vi "sv_STFT by Increment.vi"(0 "scaled signal [EU]":waveform(dbl), 1 "weighting filter":T5 items=["Linear", "A-weighting", "B-weighting", "C-weighting", "ITU-R 468-4", "Dolby", "CCITT", "C-message", "Wb", "Wc", "Wd", "We", "Wf", "Wh", "Wj", "Wk", "Wm", "AES17 20 kHz lowpass", "AES17 40 kHz lowpass", "AES17 20 kHz highpass", "AES17 40 kHz highpass"], 7 "FFT info":T7={"FFT block size"=1024, "number of FFT"=0, "start index"=0, "increment"=0.0} {"increment" format="%.2f"}, 11 "error in (no error)":errorcluster, 12 "window":T8(ring)=enum."Hanning", 13 "dB On (T)":bool=TRUE) -> (4 "power spectra [dB EU]":dbl[][](array[numeric]) format="%.2f", 6 "unit label":string, 8 "f0 and delta f [Hz]":cluster{"f0":dbl, "delta f":dbl} {"delta f" format="%.2f"; "f0" format="%.2f"}, 10 "spectrum info":T1={"channel name"="", "description"="", "x-axis units"=0, "spectral info"={"spectrum type"=enum."Power [Magnitude^2]", "linear/dB"=enum."linear", "window"=0, "window size"=0, "FFT size"=0}, "engineering units"=0, "custom label"="", "dB reference [EU]"=0.0, "peak units"=enum."rms", "weighting filter"=0, "spectral density?"=FALSE, "unit label"="", "spectrum skewed?"=FALSE, "complimentary spectrum units"=enum."none"} {"x-axis units" items=["Time (s)"=0, "Frequency-CB (Hz)"=1, "Frequency-CPB (Hz)"=1248, "Frequency-Arbitrary (Hz)"=2357, "Quefrency (s)"=2, "Revolutions (rev)"=3, "Order"=4, "Speed (RPM)"=11, "Speed (rad/s)"=21, "Index"=65535]; "weighting filter" items=["Linear", "A-weighting", "B-weighting", "C-weighting", "ITU-R 468-4", "Dolby", "CCITT", "C-message", "Wb", "Wc", "Wd", "We", "Wf", "Wh", "Wj", "Wk", "Wm", "AES17 20 kHz lowpass", "AES17 40 kHz lowpass", "AES17 20 kHz highpass", "AES17 40 kHz highpass"]; "dB reference [EU]" format="%.2f"; "engineering units" items=["custom..."=0, "V"=1, "A"=21, "C"=30, "pC"=31, "s"=32, "-"=29, "Pa"=2, "N"=20, "g"=3, "m/s^2"=4, "m/s"=5, "m"=6, "mm/s"=12, "mm"=13, "micron/s"=14, "micron"=15, "in/s^2"=7, "in/s"=8, "in"=9, "mil/s"=10, "mil"=11, "rad/s^2"=16, "rad/s"=17, "rad"=18, "deg/s^2"=26, "deg/s"=27, "deg"=28, "RPM"=22, "cycle/s^2"=23, "Hz"=24, "cycle"=25, "strain"=19]; "spectral info"."window" items=["None "=0, "Hanning"=1, "Hamming"=2, "Blackman-Harris"=3, "Exact Blackman"=4, "Blackman"=5, "Flat Top"=6, "4 Term B-Harris "=7, "7 Term B-Harris"=8, "Low Sidelobe"=9, "Force - Exponential"=10, "Gaussian"=62]}, 15 "error out":errorcluster)   [LabVIEW 2017, in "SoundVib_Transient.lvlib"]
uses:
  <vilib>/addons/Sound and Vibration/svt_Transients/SoundVib_Transient.lvlib
  <vilib>/addons/_NISVFA/_Shared subVIs/Controls/svc_Weighting Filter Text Ring.ctl
  <vilib>/addons/_NISVFA/_Shared subVIs/Controls/svc_Spectrum Info.ctl
  <vilib>/addons/_NISVFA/_Shared subVIs/Controls/svc_X-Axis Units.ctl
  <vilib>/addons/_NISVFA/_Shared subVIs/Controls/svc_Spectrum Type.ctl
  <vilib>/addons/_NISVFA/_Shared subVIs/Controls/svc_Engineering Units Text Ring.ctl
  <vilib>/addons/_NISVFA/_Shared subVIs/Controls/svc_Complimentary Spectrum Units.ctl
  <vilib>/addons/Sound and Vibration/svt_Weighting/SVT Weighting Filter (frequency) (1 Ch).vi
  <vilib>/addons/_NISVFA/_Baseband FFT/SVFA Power Spectrum (1 Ch).vi
  <vilib>/addons/Sound and Vibration/svt_Weighting/SoundVib_ABCWeighting.lvlib
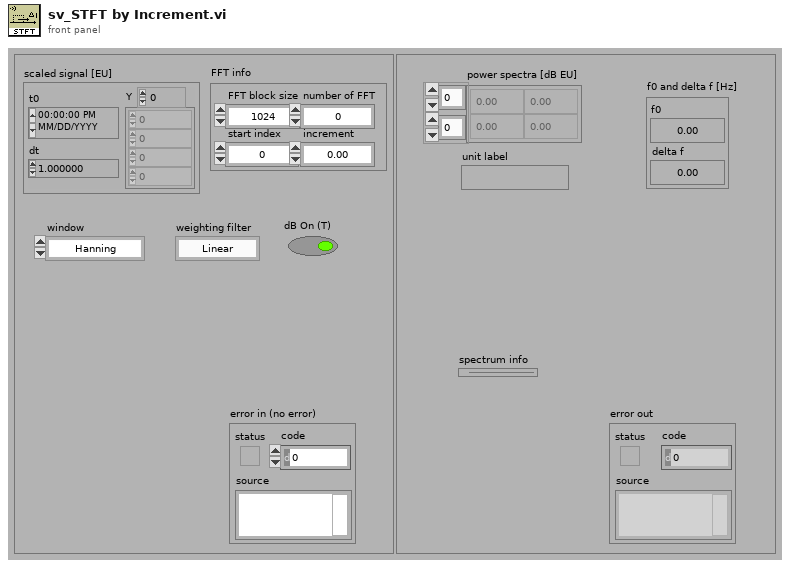
[diagram p1: front panel]
types:
  T1 = typedef "svc_Spectrum Info.ctl" = cluster{"channel name":string, "description":string, "x-axis units":T2, "spectral info":cluster{"spectrum type":T3, "linear/dB":enum16{"linear", "dB"}, "window":u16, "window size":i32, "FFT size":i32}, "engineering units":T4, "custom label":string, "dB reference [EU]":dbl, "peak units":enum16{"rms", "peak", "peak-peak"}, "weighting filter":T5, "spectral density?":bool, "unit label":string, "spectrum skewed?":bool, "complimentary spectrum units":T6}
  T2 = typedef "svc_X-Axis Units.ctl" = u16
  T3 = typedef "svc_Spectrum Type.ctl" = enum16{"FFT Spectrum [complex]", "Amplitude [Magnitude]", "Power [Magnitude^2]", "Cross Spectrum [complex]", "Frequency Response [Complex]"}
  T4 = typedef "svc_Engineering Units Text Ring.ctl" = u16
  T5 = typedef "svc_Weighting Filter Text Ring.ctl" = u16
  T6 = typedef "svc_Complimentary Spectrum Units.ctl" = enum16{"none", "radians", "degrees", "cycles", "imaginary"}
  T7 = cluster{"FFT block size":i32, "number of FFT":i32, "start index":i32, "increment":dbl}
  T8 = enum16{"None ", "Hanning", "Hamming", "Blackman-Harris", "Exact Blackman", "Blackman", "Flat Top", "4 Term B-Harris ", "7 Term B-Harris", "Low Sidelobe"}
  T9 = cluster{"averaging mode":enum16{"No averaging", "Vector averaging", "RMS averaging", "Peak hold"}, "weighting mode":enum16{"Linear", "Exponential"}, "number of averages":u32, "linear mode":enum16{"One shot", "Auto restart"}}
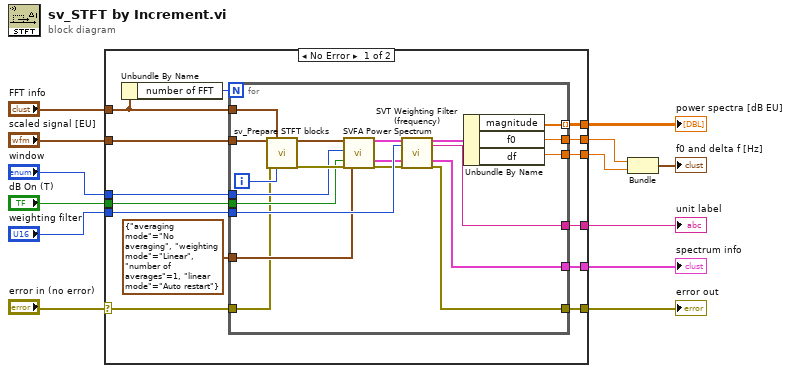
[diagram p0: block diagram]
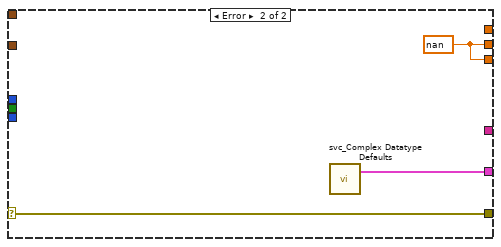
[diagram p2: hidden frame]
diagram:
  n1 = case shown="No Error" "error in (no error)" {
    selector: "error in (no error)" -> [w17 w50]
    tunnel: "dB On (T)" -> [w27 _]
    tunnel: "window" -> [w26 _]
    tunnel: "scaled signal [EU]" -> [w25 _]
    tunnel: "weighting filter" -> [w24 _]
    tunnel: [w23 _] -> w9
    tunnel: [w22 _] -> w8
    tunnel: [w21 w48] -> w7
    tunnel: "FFT info" -> [w20 _]
    tunnel: [w16 w50] -> w3
    tunnel: [w15 w48] -> w2
    tunnel: [w14 w49] -> w1
    frame No Error {
      n2 = Unbundle By Name(w20) -> ("number of FFT"=w19:i32)
      n3 = for {
        N: w19 -> [_]
        tunnel: w27 -> [w35]
        tunnel: w26 -> [w34]
        tunnel: w25 -> [w47]
        tunnel: w20 -> [w46]
        tunnel: w24 -> [w44]
        tunnel: [w43] -> w23 mode=indexing
        tunnel: [w42] -> w22
        tunnel: [w41] -> w21
        tunnel: T9 {"averaging mode"=enum."No averaging", "weighting mode"=enum."Linear", "number of averages"=1, "linear mode"=enum."Auto restart"} ("averaging parameters") -> [w33]
        tunnel: w17 -> [w32]
        tunnel: [w31] -> w16
        tunnel: [w30] -> w15
        tunnel: [w28] -> w14
        i -> [w45]
        n4 = call <vilib>:"sv_Prepare STFT blocks.vi"("scaled signal [EU]"=w47, "FFT info"=w46, "error in (no error)"=w32, "iteration"=w45) -> ("scaled signal [EU]"=w40:waveform(dbl), "error out"=w36:errorcluster)  [unwired: 10 in]
        n5 = call-poly <vilib>:"SVFA Power Spectrum.vi"("scaled signal [EU]"=w40, "window"=w34, "dB On (T)"=w35, "error in (no error)"=w36, "averaging parameters"=w33) -> ("power spectrum [dB EU]"=w39:cluster{"f0":dbl, "df":dbl, "magnitude":dbl[]}, "spectrum info"=w37:T1, "error out"=w38:errorcluster)  [unwired: 9 in, 3 out]
        n6 = call-poly <vilib>:"SVT Weighting Filter (frequency).vi"("spectrum"=w39, "weighting"=w44, "spectrum info in"=w37, "error in (no error)"=w38) -> ("weighted spectrum"=w29:cluster{"f0":dbl, "df":dbl, "magnitude":dbl[]}, "unit label"=w42:string, "spectrum info out"=w28:T1, "error out"=w31:errorcluster)  [unwired: 12 in]
        n7 = Unbundle By Name(w29) -> ("magnitude"=w43:dbl[], "f0"=w30:dbl, "df"=w41:dbl)
      }
    }
    frame Error {
      w48 = nan ("f0")
      n8 = call <vilib>:"svc_Complex Datatype Defaults.vi"() -> ("dead spectrum info"=w49:T1)  [unwired: 11 in, 8 out]
    }
  }
  "power spectra [dB EU]" <- w9
  "unit label" <- w8
  "error out" <- w3
  "spectrum info" <- w1
  n9 = Bundle("f0"=w2, "f0"=w7) -> (→"f0 and delta f [Hz]":cluster{"f0":dbl, "f0":dbl})  [unwired: 1 in]
